vi "emi_DNU Variant With Array to 1D array of Variant.vi"(0 "Array inn":variant, 11 "error in (no error)":errorcluster) -> (4 "Array Copy":variant, 6 "1D Array of Variant":variant[](array[variant]), 8 "Dimention sizes of Array":u32[](array[numeric]), 10 "Single Element TD":i16[](array[numeric]), 15 "error out":errorcluster)   [LabVIEW 2010]
doc: "Convert an array containing an array, into an array of Variants. The array of vairants will always be 1D, even if the actual aray was different dimentiens. The dimentions are published in Dimention sizes of Array. The Type def information for single elements are made available in Dingle Element TD.\n\nFIKK IKKE TIL Å BRUKE DENNE I SKRIVING/LESING AV INI FILE. TROR DEN GJØR DET DEN SKAL; MEN AT DET ER BRUKEN SOM ER FEIL:"
uses:
  Error/emi_Create Error.vi
  <vilib>/Utility/VariantDataType/GetNumericInfo.vi
  <vilib>/Utility/VariantDataType/VariantType.lvlib
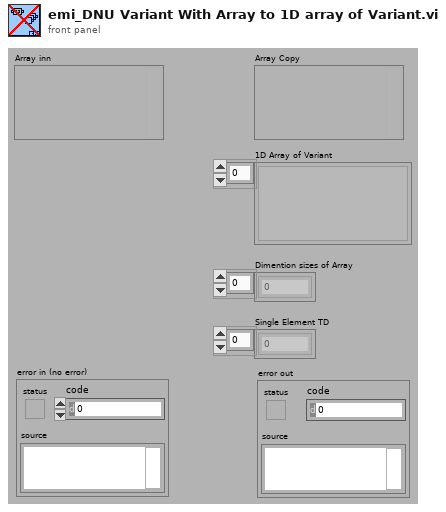
[diagram p1: front panel]
types:
  T1 = typedef "VariantType.lvlib/Type.ctl" = enum8{"Invalid Type", "Void", "I8", "I16", "I32", "I64", "U8", "U16", "U32", "U64", "Single Float", "Double Float", "Extended Float", "Single Complex", "Double Complex", "Extended Complex", "Enum U8", "Enum U16", "Enum U32", "Enum U64", "Single Float With Unit", "Double Float With Unit", "Extended Float With Unit", "Single Complex with Unit", "Double Complex with Unit", "Extended Complex with Unit", "Boolean", "String", "Path", "Picture", "Tag", "Array", "Cluster", "Variant", "LV Variant", "Waveform", "Timestamp", "Digital Waveform", "Digital Data", "ExpressData", "Refnum", "External Data", "VI", "Poly VI", "LabVIEW Class Instance", "Fixed Point"}
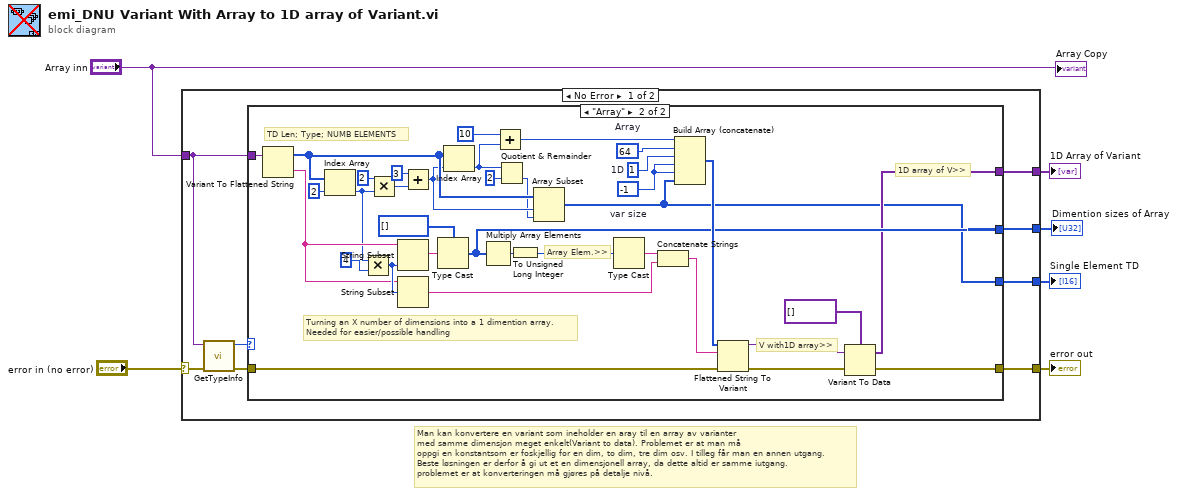
[diagram p0: block diagram]
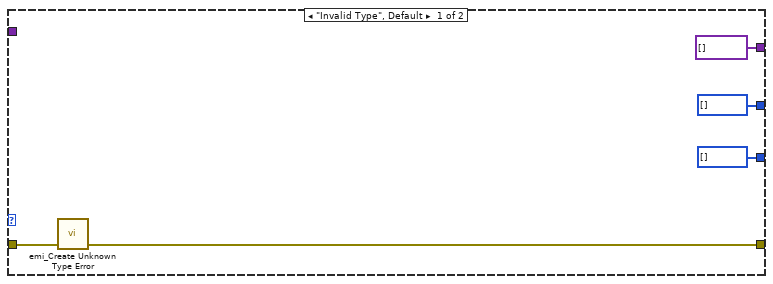
[diagram p2: hidden frame]
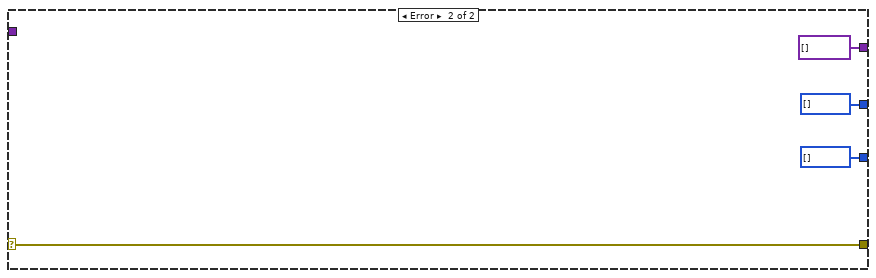
[diagram p3: hidden frame]
diagram:
  # "Man kan konvertere en variant som ineholder en aray til en array av varianter \nmed samme dimensjon meget enkelt(Variant to data). Problemet er at man må\noppgi en konstantsom er foskjellig for en dim, to dim, tre dim osv. I tilleg får man en annen utgang.\nBeste løsningen er derfor å gi ut et en dimensjonell array, da dette altid er samme iutgang.\nproblemet er at konverteringen må gjøres på detalje nivå."
  n1 = case shown="No Error" "error in (no error)" {
    selector: "error in (no error)" -> [w13 w58]
    tunnel: "Array inn" -> [w10 _]
    tunnel: [w12 w58] -> w6
    tunnel: [w9 u32[] []] -> w4
    tunnel: [w8 variant[] []] -> w5
    tunnel: [w7 i16[] []] -> w2
    frame No Error {
      n2 = call <vilib>:"GetTypeInfo.vi"("error in (no error)"=w13, "Variant"=w10) -> ("error out"=w11:errorcluster, "Type Enum"=w14:T1)  [unwired: 5 in, 3 out]
      n3 = case shown="\"Array\"" w14 {
        tunnel: w10 -> [_ w54]
        tunnel: [w18 w24] -> w12
        tunnel: w11 -> [w19 w27]
        tunnel: [u32[] [] w26] -> w9
        tunnel: [variant[] [] w21] -> w8
        tunnel: [i16[] [] w20] -> w7
        frame "Invalid Type", Default {
          n4 = call "emi_Create Unknown Type Error.vi"("error IO"=w19) -> ("error out"=w18:errorcluster)  [unwired: 14 in]
        }
        frame "Array" {
          w37 = i16 -1  # var size
          w38 = i16 1  # 1D
          w39 = i16 64  # Array
          # "1D array of V>>"
          # "V with1D array>>"
          # "Turning an X number of dimensions into a 1 dimention array.\nNeeded for easier/possible handling"
          # "Array Elem.>>"
          # "TD Len; Type; NUMB ELEMENTS"
          n5 = Variant To Flattened String(Variant=w54) -> (data string=w48:string, 1:w36:i16[])
          n6 = Index Array(array=w36, index=2) -> (element=w47:i16)
          n7 = Multiply(x=w47, y=i16 4) -> (x*y=w49:i16)
          n8 = Multiply(x=i16 2, y=w47) -> (x*y=w45:i16)
          n9 = String Subset(string=w48, length (rest)=w49) -> (substring=w51:string)  [unwired: 1 in]
          n10 = String Subset(string=w48, offset (0)=w49) -> (substring=w29:string)  [unwired: 1 in]
          n11 = Add(x=i16 3, y=w45) -> (x+y=w35:i16)
          n12 = Type Cast(type=u32[] [], x=w51) -> (*(type *) &x=w26:u32[])
          n13 = Index Array(array=w36, index=w35) -> (element=w42:i16)
          n14 = Multiply Array Elements(1:w26) -> (0:w32:u32)
          n15 = Add(x=i16 10, y=w42) -> (x+y=w40:i16)
          n16 = Quotient & Remainder(x=w42, y=u16 2) -> (floor(x/y)=w34:u16)  [unwired: 1 out]
          n17 = To Unsigned Long Integer(number=w32) -> (unsigned 32bit integer=w31:u32)
          n18 = Array Subset(array=w36, index=w35, length=w34) -> (w20:i16[])
          n19 = Type Cast(x=w31) -> (*(type *) &x=w30:string)  [unwired: 1 in]
          n20 = Concatenate Strings(w30, w29) -> (w28:string)
          n21 = Build Array (concatenate)(w40, w39, w38, w37, w37, w20) -> (w33:i16[])
          n22 = Flattened String To Variant(4:w27, 6:w28, 7:w33) -> (0:w25:errorcluster, 3:w23:variant)
          n23 = Variant To Data(error in=w25, Variant=w23, type=variant[] []) -> (error out=w24:errorcluster, data=w21:variant[])
        }
      }
    }
    frame Error {
    }
  }
  "error out" <- w6
  "1D Array of Variant" <- w5
  "Dimention sizes of Array" <- w4
  "Single Element TD" <- w2
  "Array Copy" <- "Array inn"
